vi "GSP_CF_ChangeGUI.vi"(4 "error in (no error)":errorcluster, 6 "Focus (motor counts)":i32(knob) scale=-500.0..5000.0) -> (0 "error out":errorcluster, 1 "Go?":bool, 2 "Target Out":i32)   [LabVIEW 2015]
panel:
  in  "GO":bool
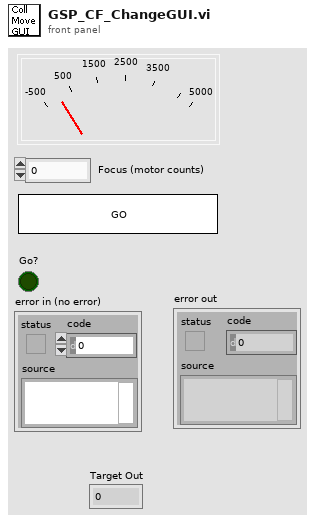
[diagram p1: front panel]
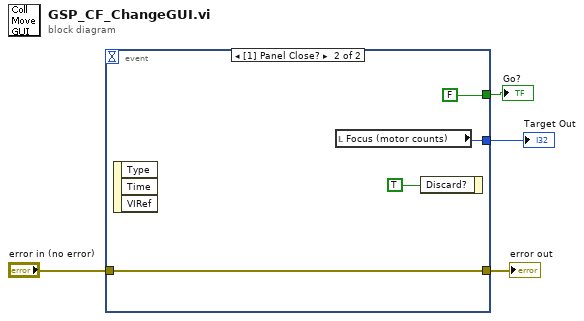
[diagram p0: block diagram]
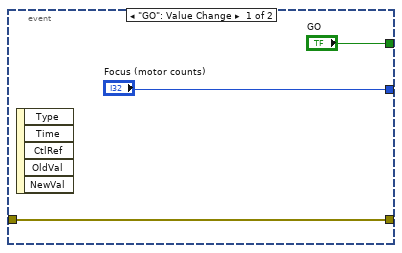
[diagram p2: hidden frame]
diagram:
  n1 = event shown="[1] Panel Close?" {
    selector: _ -> [_ _]
    dyn-events: _ -> [_ _]
    timeout: _ -> [_ _]
    tunnel: "error in (no error)" -> [w5 w10]
    tunnel: ["GO" FALSE] -> w1
    tunnel: [w5 w10] -> w3
    tunnel: ["Focus (motor counts)" w9] -> w2
    event "GO": Value Change {
      n2 = event-data() -> ()  [unwired: 1 in, 5 out]
    }
    event Panel Close? {
      n3 = event-data() -> ()  [unwired: 1 in, 3 out]
      n4 = local read "Focus (motor counts)"() -> (w9:i32)
      n5 = event-data("Discard?"=TRUE) -> ()  [unwired: 1 in, 1 out]
    }
  }
  "error out" <- w3
  "Target Out" <- w2
  "Go?" <- w1
